vi "Exercise 7.2_Elegant Answer.vi"() -> ()   [LabVIEW 2010]
panel:
  in  "stop":bool
  out "Locked/Unlocked":bool
  in  "Clear":bool
  out "Code Entered":string
  in  "Enter":bool
  in  "Button 9":bool
  in  "Button 8":bool
  in  "Button 7":bool
  in  "Button 6":bool
  in  "Button 5":bool
  in  "Button 4":bool
  in  "Button 3":bool
  in  "Button 2":bool
  in  "Button 1":bool
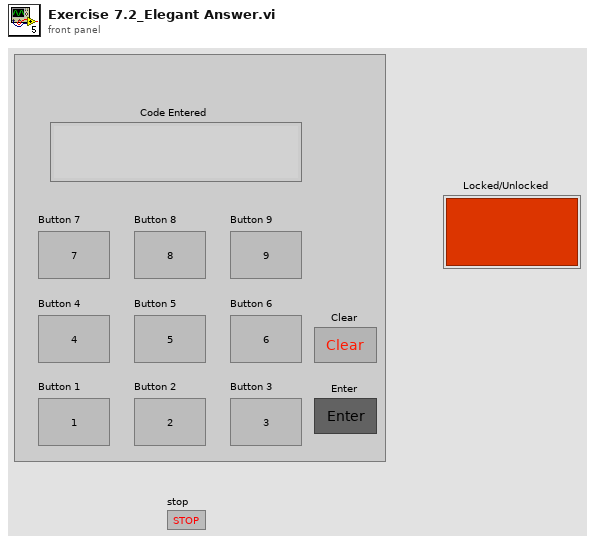
[diagram p1: front panel]
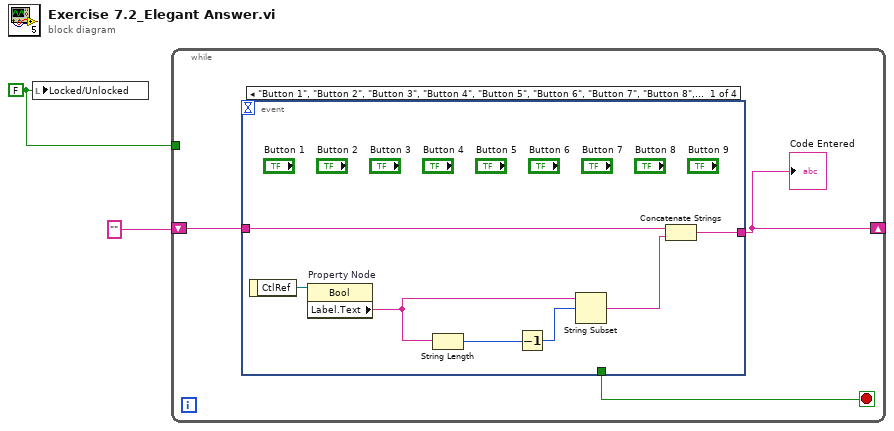
[diagram p0: block diagram]
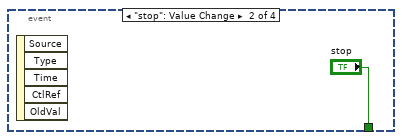
[diagram p2: hidden frame]
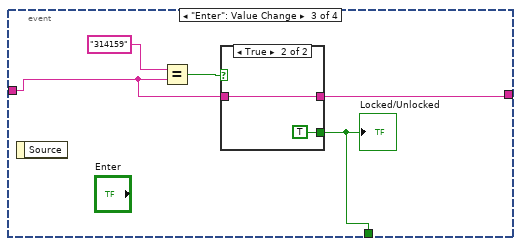
[diagram p3: hidden frame]
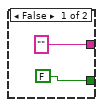
[diagram p4: hidden frame]
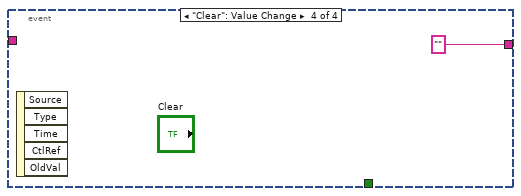
[diagram p5: hidden frame]
diagram:
  w1 = FALSE ("Locked/Unlocked")
  n1 = local write "Locked/Unlocked"(w1) -> ()
  n2 = while {
    shift-right: [w4] -> _
    shift-left: "" -> [w5]
    tunnel: w1 -> [_]
    stop <- w3 stop-if-true
    n3 = event shown="[0] \"Button 1\", \"Button 2\", \"Button 3\", \"Button 4\", \"Button 5\", \"Button 6\", \"Button 7\", \"Button 8\", \"Button 9\": Value Change" {
      selector: _ -> [_ _ _ _]
      dyn-events: _ -> [_ _ _ _]
      timeout: _ -> [_ _ _ _]
      tunnel: w5 -> [w12 _ w16 _]
      tunnel: [w11 _ w15 ""] -> w4
      tunnel: [_ "stop" w14 _] -> w3
      event "Button 1", "Button 2", "Button 3", "Button 4", "Button 5", "Button 6", "Button 7", "Button 8", "Button 9": Value Change {
        n4 = event-data() -> ("CtlRef"=w10:refnum<vi>)  [unwired: 1 in]
        n5 = property on="Property Node" class="Bool"(reference=w10) -> ("Label.Text"=w7:string)  [unwired: 1 in, 2 out]
        n6 = String Length(string=w7) -> (length=w9:i32)
        n7 = Decrement(x=w9) -> (x-1=w8:i32)
        n8 = String Subset(string=w7, offset (0)=w8) -> (substring=w6:string)  [unwired: 1 in]
        n9 = Concatenate Strings(w12, w6) -> (w11:string)
      }
      event "stop": Value Change {
        n10 = event-data() -> ()  [unwired: 1 in, 5 out]
      }
      event "Enter": Value Change {
        n11 = event-data() -> ()  [unwired: 1 in, 1 out]
        n12 = Equal?(x="314159", y=w16) -> (x = y?=w17:bool)
        n13 = case shown="True" w17 {
          tunnel: w16 -> [_ w22]
          tunnel: ["" w22] -> w15
          tunnel: [FALSE ("Locked/Unlocked") TRUE ("Locked/Unlocked")] -> w14
          frame False {
          }
          frame True {
          }
        }
        "Locked/Unlocked" <- w14
      }
      event "Clear": Value Change {
        n14 = event-data() -> ()  [unwired: 1 in, 5 out]
      }
    }
    "Code Entered" <- w4
  }
